vi "Get WAMP error details.vi"(8 "error in (no error)":errorcluster, 9 "Details Index":i32=3, 11 "WAMP Message":T3) -> (0 "error out":errorcluster, 3 "Combined Error":T1={"Error?"=FALSE, "WAMP Error"={"Error URI"="", "Error Arguments"="", "Error ArgumentKw"="{}", "Error Details"="{}"}, "Associated LabVIEW Error"={"status"=FALSE, "code"=0, "source"=""}})   [LabVIEW 2020, in "wamplv.lvlib" / "WAMP Client.lvclass"]
doc: "Gets details of a WAMP error message.\n\nNote that the output error terminal represents any errors in getting the details of the WAMP error, and not the WAMP error itself."
uses:
  WAMP Client.lvclass
  API/TypeDefs/Error or abort detail (JSON).ctl
  wamplv.lvlib
  <vilib>/ErrorRing/Error Ring.xnode
  <vilib>/Utility/error.llb/Error Cluster From Error Code.vi
  API/TypeDefs/Combined error.ctl
  7793e780-c964-3f9f-a0da-0f708762c33f.vi
  Private/TypeDefs/WAMP Message Codes.ctl
  TypeDef/WAMP Received Message_DELETE.ctl
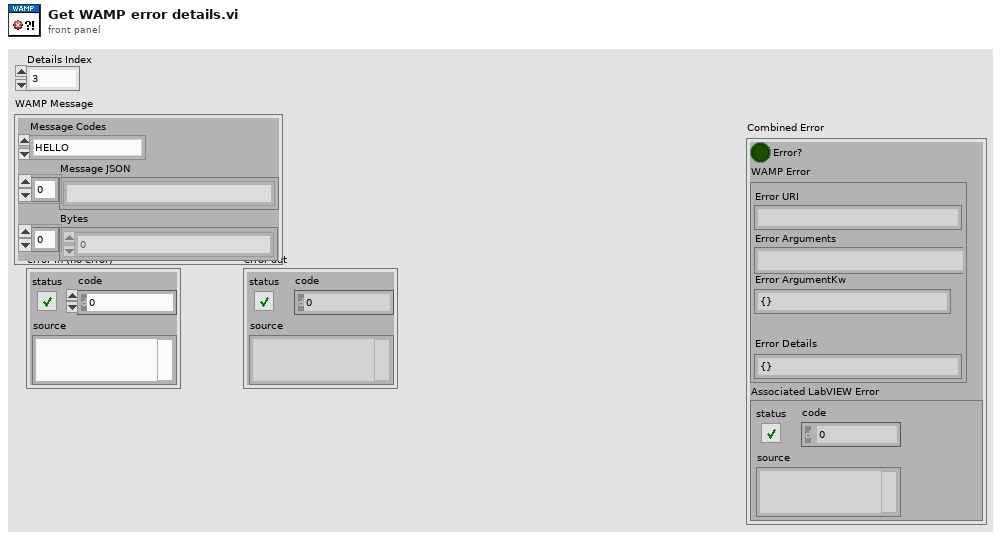
[diagram p1: front panel]
types:
  T1 = typedef "wamplv.lvlib/Combined error.ctl" = cluster{"Error?":bool, "WAMP Error":T2, "Associated LabVIEW Error":errorcluster}
  T2 = typedef "wamplv.lvlib/Error or abort detail (JSON).ctl" = cluster{"Error URI":string, "Error Arguments":string, "Error ArgumentKw":string, "Error Details":string}
  T3 = typedef "wamplv.lvlib/WAMP Client.lvclass/WAMP Received Message_DELETE.ctl" = cluster{"Message Codes":T4, "Message JSON":string[], "Bytes":u8[]}
  T4 = typedef "wamplv.lvlib/WAMP Message Codes.ctl" = enum8{"HELLO", "WELCOME", "CHALLENGE", "AUTHENTICATE", "ABORT", "GOODBYE", "ERROR", "PUBLISH", "PUBLISHED", "SUBSCRIBE", "SUBSCRIBED", "UNSUBSCRIBE", "UNSUBSCRIBED", "EVENT", "CALL", "RESULT", "REGISTER", "REGISTERED", "UNREGISTER", "UNREGISTERED", "INVOCATION", "YIELD"}
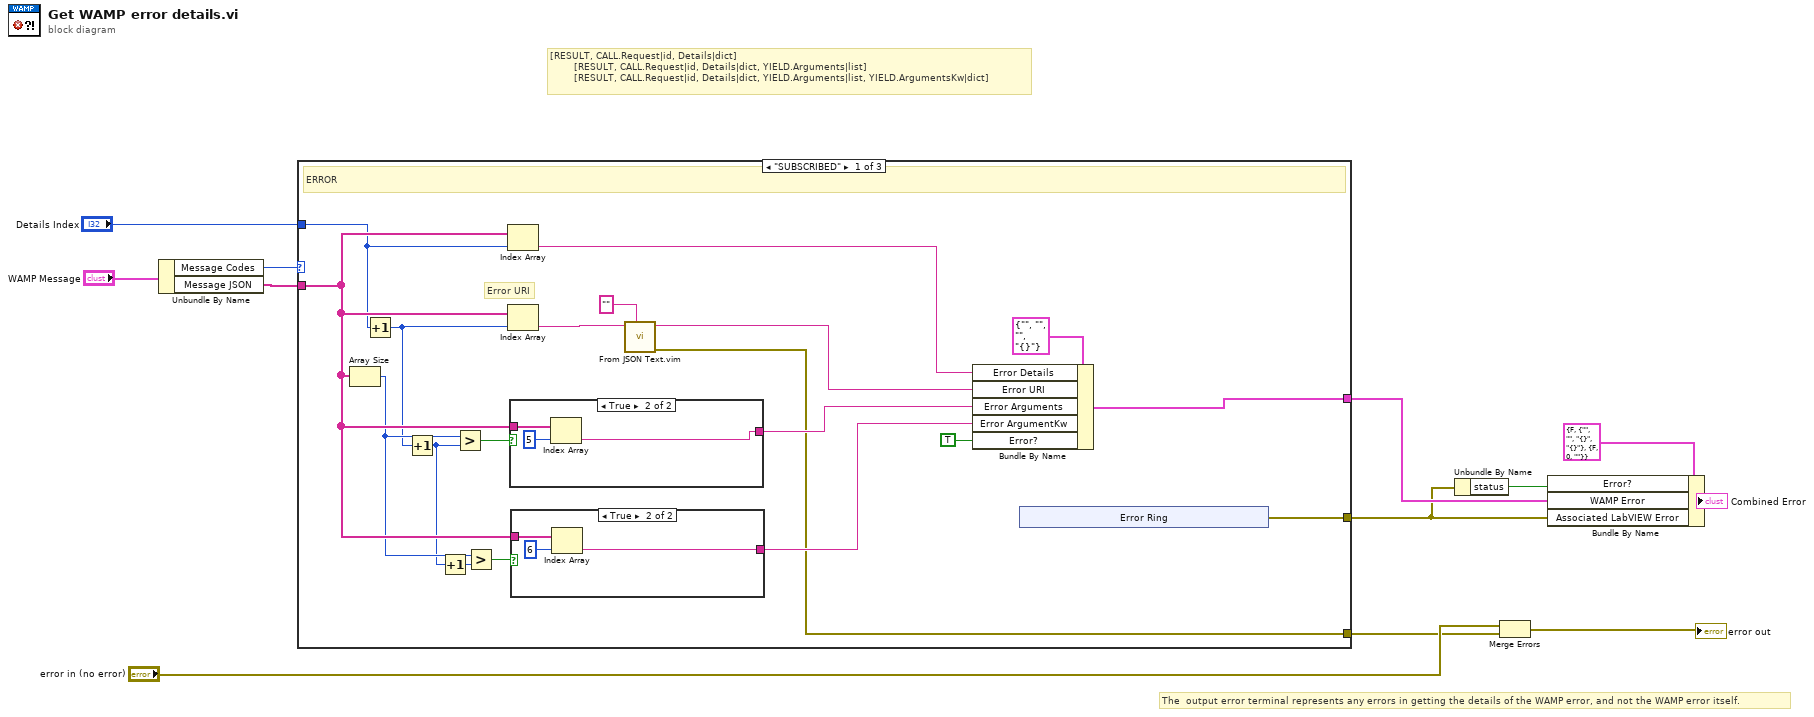
[diagram p0: block diagram]
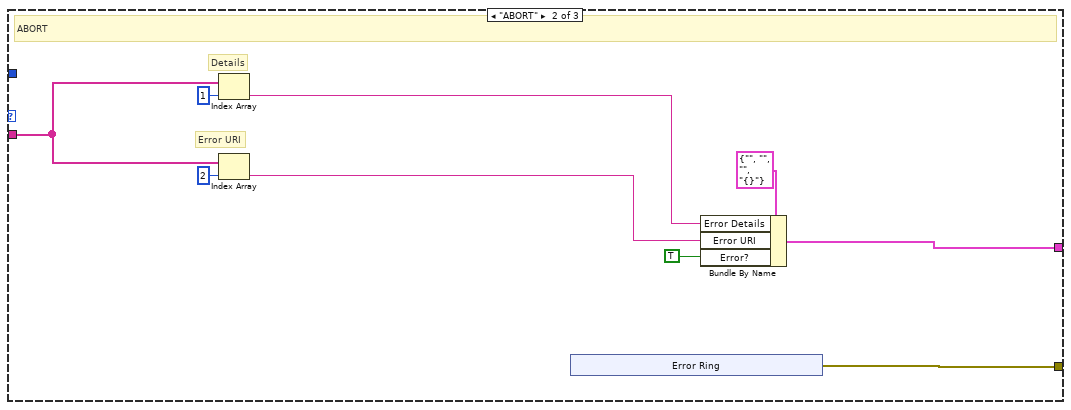
[diagram p4: hidden frame]
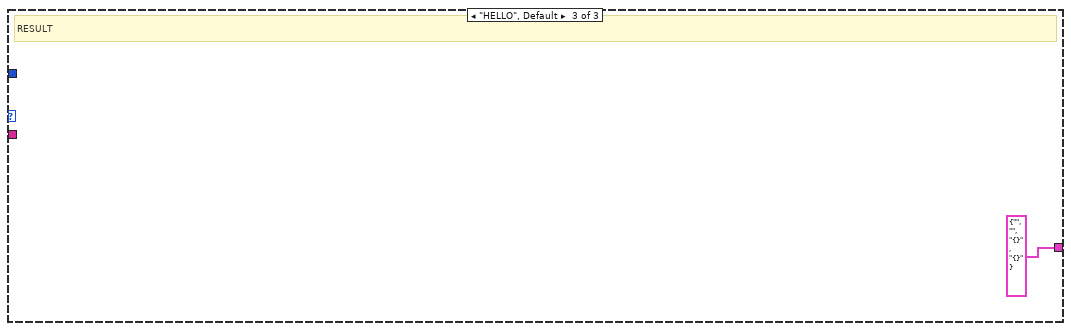
[diagram p5: hidden frame]
diagram:
  # "The  output error terminal represents any errors in getting the details of the WAMP error, and not the WAMP error itself."
  # "[RESULT, CALL.Request|id, Details|dict]\n        [RESULT, CALL.Request|id, Details|dict, YIELD.Arguments|list]\n        [RESULT, CALL.Request|id, Details|dict, YIELD.Arguments|list, YIELD.ArgumentsKw|dict]"
  n1 = Unbundle By Name("WAMP Message") -> ("Message Codes"=w11:T4, "Message JSON"=w10:string[])
  n2 = case shown="\"SUBSCRIBED\"" w11 {
    tunnel: w10 -> [w30 w50 _]
    tunnel: [w15 w42 _] -> w6
    tunnel: [w25 w47 T2 {"Error URI"="", "Error Arguments"="", "Error ArgumentKw"="{}", "Error Details"="{}"} ("Cluster")] -> w7
    tunnel: "Details Index" -> [w23 _ _]
    tunnel: [w14 _ _] -> w2
    frame "SUBSCRIBED" {
      # "Error URI"
      # "ERROR"
      n3 = Array Size(array=w30) -> (size(s)=w28:i32)
      n4 = Increment(x=w23) -> (x+1=w22:i32)
      n5 = Increment(x=w22) -> (x+1=w20:i32)
      n6 = Increment(x=w20) -> (x+1=w21:i32)
      n7 = Greater?(x=w28, y=w20) -> (0:w31:bool)
      n8 = Greater?(x=w28, y=w21) -> (0:w29:bool)
      n9 = Index Array(array=w30, index=w23) -> (element=w19:string)
      n10 = Index Array(array=w30, index=w22) -> (element=w18:string)
      n11 = case shown="True" w31 {
        tunnel: w30 -> [_ w40]
        tunnel: [_ w39] -> w24
        frame False {
        }
        frame True {
          n12 = Index Array(array=w40, index=5) -> (element=w39:string)
        }
      }
      n13 = case shown="True" w29 {
        tunnel: [_ w37] -> w26
        tunnel: w30 -> [_ w36]
        frame False {
        }
        frame True {
          n14 = Index Array(array=w36, index=6) -> (element=w37:string)
        }
      }
      n15 = call "From JSON Text.vim"("Data Type and Default Value"="", "JSON"=w18) -> ("error out"=w14:errorcluster, "Data out"=w16:string)  [unwired: 8 in]
      n16 = Bundle By Name(cluster=T2 {"Error URI"="", "Error Arguments"="", "Error ArgumentKw"="", "Error Details"="{}"} ("Cluster"), "Error Details"=w19, "Error URI"=w16, "Error Arguments"=w24, "Error ArgumentKw"=w26, "Error?"=TRUE) -> (w25:T2)
      n17 = xnode "Error Ring"() -> ("error out"=w15:errorcluster)
    }
    frame "ABORT" {
      # "Details"
      # "Error URI"
      # "ABORT"
      n18 = Index Array(array=w50, index=1) -> (element=w45:string)
      n19 = Index Array(array=w50, index=2) -> (element=w46:string)
      n20 = xnode "Error Ring"() -> ("error out"=w42:errorcluster)
      n21 = Bundle By Name(cluster=T2 {"Error URI"="", "Error Arguments"="", "Error ArgumentKw"="", "Error Details"="{}"} ("Cluster"), "Error Details"=w45, "Error URI"=w46, "Error?"=TRUE ("status")) -> (w47:T2)
    }
    frame "HELLO", Default {
      # "RESULT"
    }
  }
  n22 = Unbundle By Name(w6) -> ("status"=w5:bool)
  n23 = Merge Errors("error in (no error)", w2) -> (→"error out":errorcluster)
  n24 = Bundle By Name(cluster=T1 {"Error?"=FALSE, "WAMP Error"={"Error URI"="", "Error Arguments"="", "Error ArgumentKw"="{}", "Error Details"="{}"}, "Associated LabVIEW Error"={"status"=FALSE, "code"=0, "source"=""}} ("Combined Error"), "Error?"=w5, "WAMP Error"=w7, "Associated LabVIEW Error"=w6) -> (→"Combined Error":T1)
